vi "Simple Grabber Manager.vi"(10 "Setpoint":dbl) -> ()   [LabVIEW 2014]
uses:
  Robot Global Data.vi
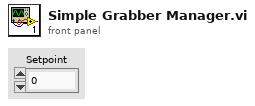
[diagram p1: front panel]
types:
  T1 = typedef "WPI_EncoderDevRef.ctl" = cluster{"DevStatus":errorcluster, "EncoderIndex":T2, "CounterIndex":T3, "DistancePerCount":dbl, "Decoding Type":T4}
  T2 = typedef "FPGA_EncoderIdx.ctl" = enum8{"Enc 0", "Enc 1", "Enc 2", "Enc 3", "Enc 4", "Enc 5", "Enc 6", "Enc 7", "Invalid"}
  T3 = typedef "FPGA_CounterCtrSystemIndex.ctl" = enum8{"Ctr 0", "Ctr 1", "Ctr 2", "Ctr 3", "Ctr 4", "Ctr 5", "Ctr 6", "Ctr 7", "Invalid"}
  T4 = typedef "WPI_EncoderType.ctl" = enum16{"1x", "2x", "4x"}
  T5 = typedef "WPI_DigitalInputDevRef.ctl" = cluster{"DevStatus":errorcluster, "DIO Channel":T6, "Controller":T7}
  T6 = typedef "FPGA_DIOChannel.ctl" = enum8{"DIO 0", "DIO 1", "DIO 2", "DIO 3", "DIO 4", "DIO 5", "DIO 6", "DIO 7", "DIO 8", "DIO 9", "DIO MXP 0", "DIO MXP 1", "DIO MXP 2", "DIO MXP 3", "DIO MXP 4", "DIO MXP 5", "DIO MXP 6", "DIO MXP 7", "DIO MXP 8", "DIO MXP 9", "DIO MXP 10", "DIO MXP 11", "DIO MXP 12", "DIO MXP 13", "DIO MXP 14", "DIO MXP 15", "Invalid"}
  T7 = typedef "FPGA_TypedefDigitalModule.ctl" = enum16{"Controller 1"}
  T8 = typedef "WPI_MotorControlDeviceRef.ctl" = cluster{"DeviceStatus":errorcluster, "Type":T9, "PWM":cluster{"Controller":T7, "PWM Channel":T10, "DeadBand":T11}, "CAN":cluster{"Device Number":u8, "Control Mode":T12, "Semaphore":T13, "Max Vout":dbl, "TalonSRX Control Mode":T14}, "Invert":bool, "TransformRef":T15, "InvTransformRef":T15}
  T9 = typedef "WPI_MotorControlType.ctl" = enum16{"PWM", "CAN", "CANTalonSRX"}
  T10 = typedef "FPGA_DIOPWMChannel.ctl" = enum8{"PWM 0", "PWM 1", "PWM 2", "PWM 3", "PWM 4", "PWM 5", "PWM 6", "PWM 7", "PWM 8", "PWM 9", "PWM MXP 0", "PWM MXP 1", "PWM MXP 2", "PWM MXP 3", "PWM MXP 4", "PWM MXP 5", "PWM MXP 6", "PWM MXP 7", "PWM MXP 8", "PWM MXP 9", "Invalid"}
  T11 = typedef "WPI_PWMDeadband.ctl" = cluster{"Name":string, "maxPositivePwm":i32, "minPositivePwm":i32, "centerPwm":i32, "maxNegativePwm":i32, "minNegativePwm":i32, "angularRange":u16}
  T12 = typedef "WPI_CANJaguar_ControlMode.ctl" = enum8{"Percent VBus", "Current", "Speed", "Position", "Voltage"}
  T13 = typedef "Semaphore RefNum" = refnum<k1>
  T14 = typedef "WPI_CANTalonSRX_APIControlMode.ctl" = enum8{"Percent VBus", "Speed", "Position", "Slave", "Unchanged / Invalid"}
  T15 = typedef "WPI_PWMTransform_ConPane.ctl" = refnum<vi>
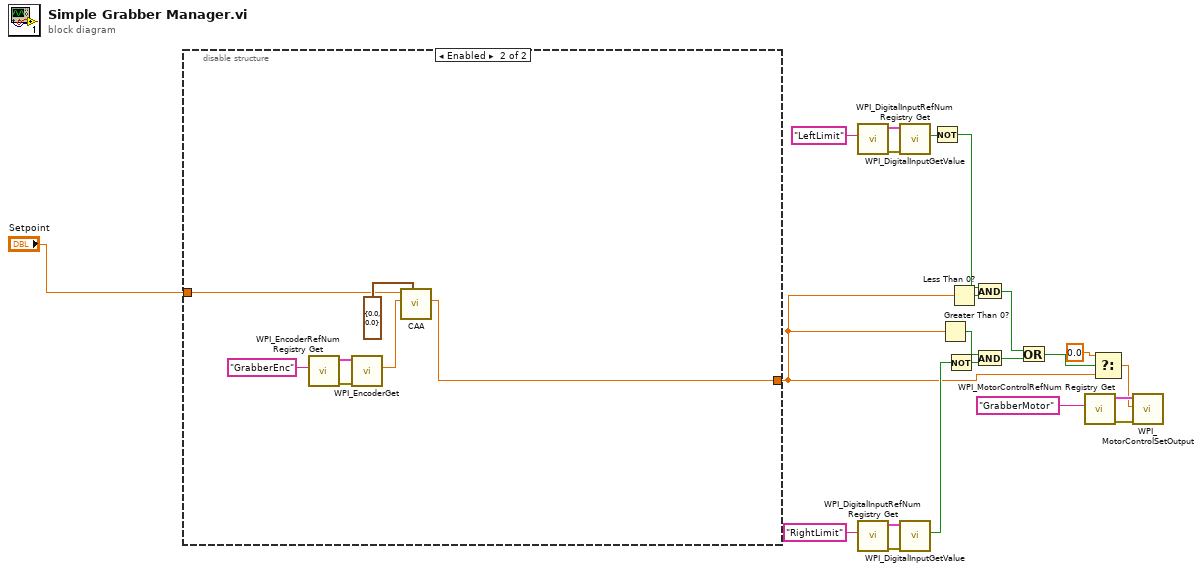
[diagram p0: block diagram]
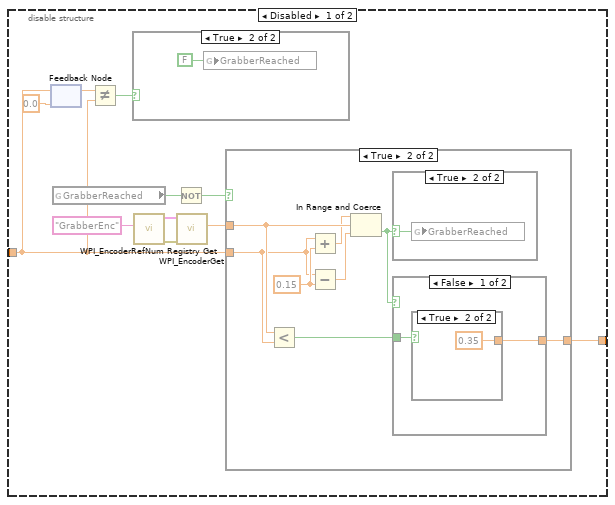
[diagram p2: hidden frame]
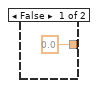
[diagram p3: hidden frame]
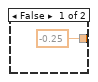
[diagram p5: hidden frame]
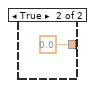
[diagram p6: hidden frame]
diagram:
  n1 = disable-structure shown="Enabled" {
    disable-tunnel: [w24 w51] -> w3
    disable-tunnel: "Setpoint" -> [w23 w55]
    frame Disabled {
      n2 = feedback #1(0.0) -> (w28:dbl)
      n3 = feedback-in #1(w23) -> ()
      n4 = global read "Robot Global Data.vi" "GrabberReached"() -> (w26:bool)
      n5 = Not Equal?(x=w28, y=w23) -> (x != y?=w27:bool)
      n6 = case shown="True" w27 {
        frame False {
        }
        frame True {
          n7 = global write "Robot Global Data.vi" "GrabberReached"(FALSE) -> ()
        }
      }
      n8 = call <vilib>:"WPI_EncoderRefNum Registry Get.vi"("refnum name"="GrabberEnc") -> ("error out"=w32:errorcluster, "EncoderDevRef"=w31:T1)  [unwired: 9 in]
      n9 = Not(x=w26) -> (.not. x?=w25:bool)
      n10 = call <vilib>:"WPI_EncoderGet.vi"("error in (no error)"=w32, "EncoderDevRef"=w31) -> ("Distance"=w30:dbl)  [unwired: 4 in, 5 out]
      n11 = case shown="True" w25 {
        tunnel: [0.0 w42] -> w24
        tunnel: w30 -> [_ w40]
        tunnel: w23 -> [_ w35]
        frame False {
        }
        frame True {
          w37 = 0.15
          n12 = Less?(x=w40, y=w35) -> (x < y?=w41:bool)
          n13 = Add(x=w35, y=w37) -> (x+y=w39:dbl)
          n14 = Subtract(x=w35, y=w37) -> (x-y=w38:dbl)
          n15 = In Range and Coerce(upper limit=w39, x=w40, lower limit=w38) -> (In Range?=w36:bool)  [unwired: 1 out]
          n16 = case shown="True" w36 {
            selector: w36 -> [_ w43]
            frame False {
            }
            frame True {
              n17 = global write "Robot Global Data.vi" "GrabberReached"(w43) -> ()
            }
          }
          n18 = case shown="False" w36 {
            tunnel: [w44 0.0] -> w42
            tunnel: w41 -> [w45 _]
            frame False {
              n19 = case shown="True" w45 {
                tunnel: [-0.25 0.35] -> w44
                frame False {
                }
                frame True {
                }
              }
            }
            frame True {
            }
          }
        }
      }
    }
    frame Enabled {
      n20 = call <vilib>:"WPI_EncoderRefNum Registry Get.vi"("refnum name"="GrabberEnc") -> ("error out"=w53:errorcluster, "EncoderDevRef"=w50:T1)  [unwired: 9 in]
      n21 = call <vilib>:"WPI_EncoderGet.vi"("error in (no error)"=w53, "EncoderDevRef"=w50) -> ("Distance"=w52:dbl)  [unwired: 4 in, 5 out]
      n22 = call "CAA.vi"("Levels"=cluster{"Max -> Mid":dbl, "Mid -> Min":dbl} {"Max -> Mid"=0.0, "Mid -> Min"=0.0}, "Process Variable"=w52, "Setpoint"=w55) -> ("Output"=w51:dbl)  [unwired: 8 in]
    }
  }
  n23 = call <vilib>:"WPI_DigitalInputRefNum Registry Get.vi"("refnum name"="LeftLimit") -> ("error out"=w14:errorcluster, "DigitalInputDevRef"=w13:T5)  [unwired: 9 in]
  n24 = call <vilib>:"WPI_DigitalInputRefNum Registry Get.vi"("refnum name"="RightLimit") -> ("error out"=w12:errorcluster, "DigitalInputDevRef"=w11:T5)  [unwired: 9 in]
  n25 = call <vilib>:"WPI_DigitalInputGetValue.vi"("error in (no error)"=w14, "DigitalInputDevRef"=w13) -> ("Value"=w7:bool)  [unwired: 7 in, 2 out]
  n26 = call <vilib>:"WPI_DigitalInputGetValue.vi"("error in (no error)"=w12, "DigitalInputDevRef"=w11) -> ("Value"=w4:bool)  [unwired: 7 in, 2 out]
  n27 = Not(x=w7) -> (.not. x?=w6:bool)
  n28 = Greater Than 0?(x=w3) -> (x > 0?=w17:bool)
  n29 = Not(x=w4) -> (.not. x?=w5:bool)
  n30 = Less Than 0?(x=w3) -> (x < 0?=w2:bool)
  n31 = And(x=w6, y=w2) -> (x .and. y?=w16:bool)
  n32 = And(x=w17, y=w5) -> (x .and. y?=w15:bool)
  n33 = Or(x=w16, y=w15) -> (x .or. y?=w19:bool)
  n34 = call <vilib>:"WPI_MotorControlRefNum Registry Get.vi"("refnum name"="GrabberMotor") -> ("error out"=w21:errorcluster, "MotorControlDevRef"=w20:T8)  [unwired: 9 in]
  n35 = Select(t=0.0, s=w19, f=w3) -> (s? t:f=w8:dbl)
  n36 = call <vilib>:"WPI_MotorControlSetOutput.vi"("error in (no error)"=w21, "Output"=w8, "MotorControlDevRef"=w20) -> ()  [unwired: 6 in, 3 out]
